vi "FTW-CodeGen-GenerateCode.vi"(0 "State In":T2, 5 "XRef":refnum<vi>, 7 "Terms":T1(array[cluster]), 9 "Diagram":refnum<vi>) -> (4 "State Out":T2, 6 "Reply":string[](array[string]), 8 "Generated Code?":bool)   [LabVIEW 2015, in "FTW-SQLite-Fetch.xnode"]
uses:
  FTW-SQLite-Fetch.xnode
  FTW-CodeGen-State.ctl
  FTW-CodeGen-XNodeReplyType.ctl
  src/reflection/FTW-Reflection-Types.ctl
  src/reflection/FTW-Reflection-Array.vi
  src/regex/FTW-Regex-Execute.vi
  src/error/FTW-ERR-ThrowGenericError.vi
  src/error/FTW-ERR-ThrowError.vi
  src/error/FTW-ERR-CallChain.vi
  src/error/FTW-ERR-NoErrorConstant.vi
  src/string/FTW-STR-ReplaceWhitespace.vi
  src/string/FTW-STR-Array-Delimit.vi
  src/regex/FTW-Regex-Construct.vi
  lib/FTW-KernelFilepath.vi
  src/regex/FTW-Regex-Destroy.vi
panel:
  # "Inputs"
  # "Outputs"
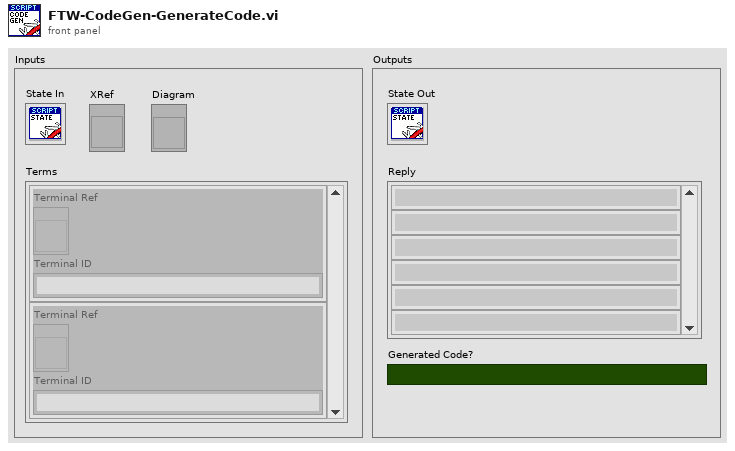
[diagram p1: front panel]
types:
  T1 = cluster{"Terminal Ref":refnum<vi>, "Terminal ID":string}[]
  T2 = typedef "FTW-SQLite-Fetch.xnode/FTW-CodeGen-State.ctl" = cluster{"Dummy":i32}
  T3 = typedef "FTW-CodeGen-XNodeReplyType.ctl" = enum16{"UpdateState", "AdaptToInputs", "AdaptAndAugment", "CosmeticUpdate", "NoReply"}
  T4 = typedef "FTW-Reflection-Types.ctl" = enum16{"Unknown", "Void", "Array", "Cluster", "LVObject", "Boolean", "I8", "I16", "I32", "I64", "U8", "U16", "U32", "U64", "SGL", "DBL", "EXT", "CSG", "CDB", "CXT", "FXP", "EnumU8", "EnumU16", "EnumU32", "EnumU64", "SGLwithUnit", "DBLwithUnit", "EXTwithUnit", "CSGwithUnit", "CDBwithUnit", "CXTwithUnit", "String", "Path", "Picture", "Tag", "LVVariant", "Timestamp", "WaveformI8", "WaveformI16", "WaveformI32", "WaveformI64", "WaveformU8", "WaveformU16", "WaveformU32", "WaveformU64", "WaveformSGL", "WaveformDBL", "WaveformEXT", "WaveformCSG", "WaveformCDB", "WaveformCXT", "WaveformDigital", "WaveformUnknownType", "DigitalData", "DynamicData", "ExternalData", "FileByteStream", "TDMStream", "dotNET", "ActiveX", "VIServerReference", "VIReference", "ApplicationInstance", "Menu", "ConnectionDataSocket", "ConnectionVISA", "ConnectionBluetooth", "ConnectionIrDA", "ConnectionTCP", "ConnectionUDP", "ConnectionHTTPClient", "ConnectionFTP", "Occurrence", "Notifier", "Queue", "Rendezvous", "Semaphore", "RTFIFO", "EventPublisher", "EventRegistration", "EventCallback", "DataValueReference", "GenericClass", "GenericClassTag", "GenericClassDeepCopy", "GenericClassFlattened", "GenericClassTagFlattened", "GenericReferenceType", "WindowsRegistry", "OverloadedDatalogRef", "ReferenceUnknownType", "ByteArray", "ConPaneInterface"}
  T5 = cluster{"Element Name":string, "Element Type":T4, "Element Value":variant}
  T6 = cluster{"Element Name":string, "Element Type":T4, "Element Value":variant}[]
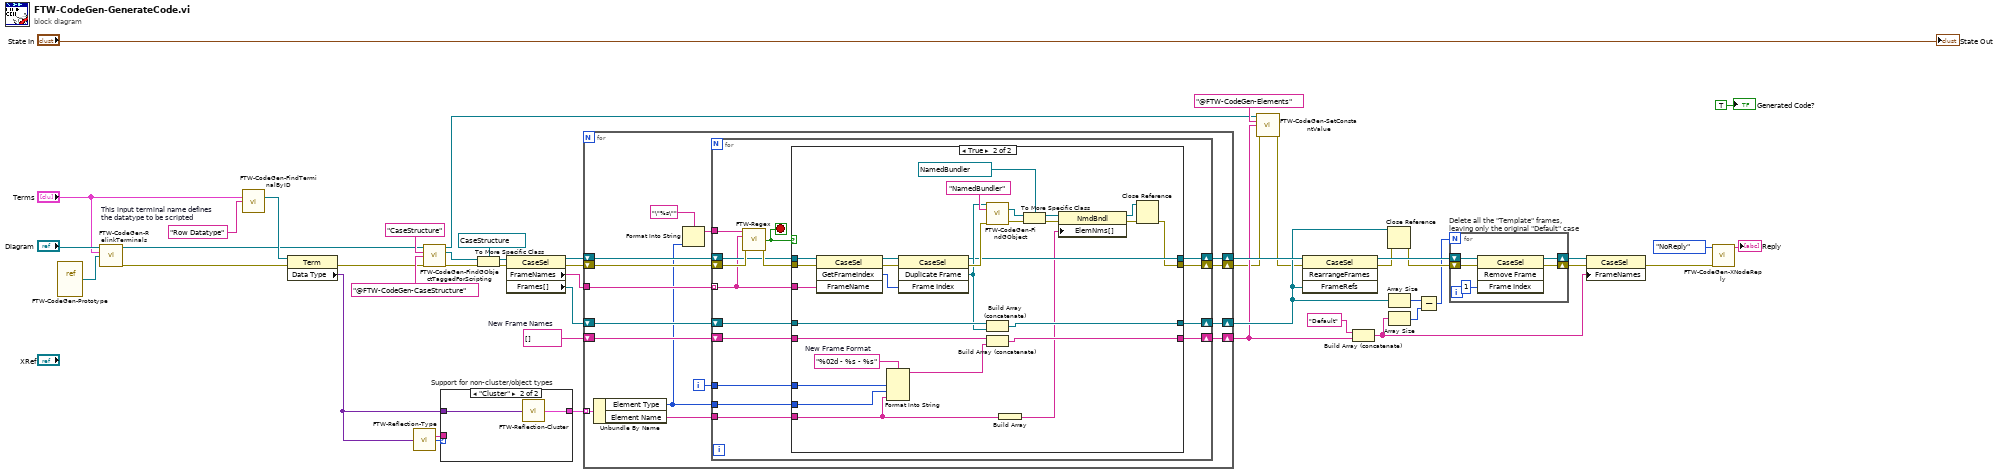
[diagram p0: block diagram]
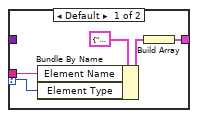
[diagram p2: hidden frame]
diagram:
  w31 = string[] []  # New Frame Names
  w9 = "Row Datatype"  # This input terminal name defines the datatype to be scripted
  n1 = vi-ref "FTW-CodeGen-Prototype.vi"() -> (w12:refnum<vi>)
  n2 = call "FTW-CodeGen-RelinkTerminals.vi"("Diagram"="Diagram", "Terms"="Terms", "PrototypeVI"=w12) -> ("Diagram out"=w5:refnum<vi>, "error out"=w16:errorcluster)  [unwired: 11 in]
  n3 = call "FTW-CodeGen-FindTerminalByID.vi"("Terms"="Terms", "Terminal ID"=w9) -> ("Terminal Ref"=w8:refnum<vi>)  [unwired: 12 in, 1 out]
  n4 = property class="Term"(reference=w8, error in=w16) -> (error out=w15:errorcluster, "Data Type"=w18:variant)  [unwired: 1 out]
  n5 = call "FTW-Reflection-Type.vi"("Anything"=w18) -> ("Data Name"=w17:string, "LabVIEW Type"=w19:T4)  [unwired: 12 in, 1 out]
  n6 = call "FTW-CodeGen-FindGObjectTaggedForScripting.vi"("GObject to Traverse"=w5, "Class Name"="CaseStructure", "Label Prefix to uniquely identify node"="@FTW-CodeGen-CaseStructure" ("Label to uniquely identify node"), "error in"=w15) -> ("GObject to Traverse out"=w4:refnum<vi>, "GObject"=w43:refnum<vi>, "error out"=w42:errorcluster)  [unwired: 9 in]
  n7 = case "Support for non-cluster/object types" shown="\"Cluster\"" w19 {
    selector: w19 -> [w47 _]
    tunnel: [w51 w53] -> w40
    tunnel: w18 -> [_ w52]
    tunnel: w17 -> [w48 _]
    frame Default {
      n8 = Bundle By Name(cluster=T5 {"Element Name"="", "Element Type"=enum."Unknown", "Element Value"=variant} ("Element"), "Element Name"=w48, "Element Type"=w47) -> (w49:T5)
      n9 = Build Array(w49) -> (w51:T6)
    }
    frame "Cluster" {
      n10 = call "FTW-Reflection-Cluster.vi"("Cluster"=w52) -> ("Cluster Elements"=w53:T6)  [unwired: 14 in]
    }
  }
  n11 = To More Specific Class(target class=refnum<vi> refnum ("Object"), reference=w43, error in=w42) -> (specific class reference=w39:refnum<vi>, error out=w37:errorcluster)
  n12 = property class="CaseSel"(reference=w39, error in=w37) -> (reference out=w38:refnum<vi>, error out=w36:errorcluster, "FrameNames"=w35:string[], "Frames[]"=w25:refnum<vi>[])
  n13 = for {
    tunnel: w40 -> [w65] mode=indexing
    tunnel: w35 -> [w66]
    shift-right: [w60] -> w29
    shift-left: w38 -> [w68]
    shift-right: [w61] -> w3
    shift-left: w36 -> [w67]
    shift-right: [w59] -> w24
    shift-left: w25 -> [w62]
    shift-right: [w57] -> w6
    shift-left: w31 -> [w58]
    i -> [w54]
    n14 = Unbundle By Name(w65) -> ("Element Type"=w55:T4, "Element Name"=w56:string)
    n15 = Format Into String(format string="\"%s\"", w55) -> (resulting string=w63:string)  [unwired: 2 in, 1 out]
    n16 = for {
      tunnel: w66 -> [w73] mode=indexing
      tunnel: w63 -> [w69]
      shift-right: [w77] -> w60
      shift-left: w68 -> [w81]
      shift-right: [w79] -> w59
      shift-left: w62 -> [w80]
      shift-right: [w78] -> w61
      shift-left: w67 -> [w83]
      shift-right: [w74] -> w57
      shift-left: w58 -> [w75]
      tunnel: w56 -> [w72]
      tunnel: w55 -> [w71]
      tunnel: w54 -> [w70]
      stop <- w76 stop-if-true
      n17 = call "FTW-Regex.vi"("Regular Expression"=w69, "Input String"=w73, "error in"=w83) -> ("Match Found?"=w76:bool, "error out"=w82:errorcluster)  [unwired: 8 in, 3 out]
      n18 = case shown="True" w76 {
        tunnel: w82 -> [w86 w110]
        tunnel: w81 -> [w87 w111]
        tunnel: w80 -> [w85 w115]
        tunnel: [w85 w112] -> w79
        tunnel: [w86 w88] -> w78
        tunnel: [w87 w95] -> w77
        tunnel: w75 -> [w84 w114]
        tunnel: [w84 w113] -> w74
        tunnel: w73 -> [_ w106]
        tunnel: w72 -> [_ w92]
        tunnel: w71 -> [_ w91]
        tunnel: w70 -> [_ w90]
        frame False {
        }
        frame True {
          w93 = "%02d - %s - %s"  # New Frame Format
          n19 = invoke class="CaseSel" method="GetFrameIndex"(reference=w111, error in=w110, "FrameName"=w106) -> (reference out=w109:refnum<vi>, error out=w108:errorcluster, "GetFrameIndex"=w107:i32)  [unwired: 1 in, 1 out]
          n20 = Format Into String(format string=w93, w90, w91, w92) -> (resulting string=w94:string)  [unwired: 2 in, 1 out]
          n21 = invoke class="CaseSel" method="Duplicate Frame"(reference=w109, error in=w108, "Frame Index"=w107) -> (reference out=w95:refnum<vi>, error out=w97:errorcluster, "Duplicate Frame"=w96:refnum<vi>)  [unwired: 1 in, 1 out]
          n22 = call "FTW-CodeGen-FindGObject.vi"("GObject to Traverse"=w96, "Class Name"="NamedBundler", "error in"=w97) -> ("GObject"=w99:refnum<vi>, "error out"=w100:errorcluster)  [unwired: 11 in]
          n23 = Build Array (concatenate)(w115, w96) -> (w112:refnum<vi>[])
          n24 = Build Array (concatenate)(w114, w94) -> (w113:string[])
          n25 = Build Array(w92) -> (w89:string[])
          n26 = To More Specific Class(target class=refnum<vi> refnum ("Object"), reference=w99, error in=w100) -> (specific class reference=w103:refnum<vi>, error out=w102:errorcluster)
          n27 = property class="NmdBndl"(reference=w103, error in=w102, "ElemNms[]"=w89) -> (reference out=w105:refnum<vi>, error out=w104:errorcluster)
          n28 = Close Reference(reference=w105, error in (no error)=w104) -> (error out=w88:errorcluster)
        }
      }
    }
  }
  n29 = call "FTW-CodeGen-SetConstantValue.vi"("GObject to Traverse"=w4, "Constant Label"="@FTW-CodeGen-Elements" ("Label to uniquely identify node"), "Value"=w6, "error in"=w3) -> ("error out"=w2:errorcluster)  [unwired: 10 in, 1 out]
  n30 = invoke class="CaseSel" method="RearrangeFrames"(reference=w29, error in=w2, "FrameRefs"=w24) -> (reference out=w28:refnum<vi>, error out=w27:errorcluster)  [unwired: 1 in, 2 out]
  n31 = Build Array (concatenate)("Default", w6) -> (w23:string[])
  n32 = Close Reference(reference=w24, error in (no error)=w27) -> (error out=w26:errorcluster)
  n33 = Array Size(array=w24) -> (size(s)=w22:i32)
  n34 = Array Size(array=w23) -> (size(s)=w21:i32)
  n35 = Subtract(x=w22, y=w21) -> (x-y=w20:i32)
  n36 = for "Delete all the \"Template\" frames,\nleaving only the original \"Default\" case" {
    N: w20 -> [_]
    shift-right: [w117] -> w33
    shift-left: w26 -> [w118]
    shift-right: [w119] -> w34
    shift-left: w28 -> [w120]
    n37 = invoke class="CaseSel" method="Remove Frame"(reference=w120, error in=w118, "Frame Index"=u32 1) -> (reference out=w119:refnum<vi>, error out=w117:errorcluster)  [unwired: 1 in, 2 out]
  }
  n38 = property class="CaseSel"(reference=w34, error in=w33, "FrameNames"=w23) -> (error out=w1:errorcluster)  [unwired: 1 out]
  n39 = call "FTW-CodeGen-XNodeReply.vi"("XNode Reply Type"=FTW-CodeGen-XNodeReplyType."NoReply", "error in"=w1) -> ("Reply"=→"Reply":string[])  [unwired: 13 in]
  "State Out" <- "State In"
  "Generated Code?" <- TRUE ("Generated Code?")
